vi "refNewton Ralphson Zero Finder.vi"   [LabVIEW 2012, in "NI_Gmath.lvlib"]
uses:
  NI_Gmath.lvlib
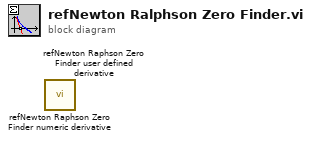
[diagram p0: block diagram]
diagram:
  n1 = call "refNewton Raphson Zero Finder numeric derivative.vi"() -> ()  [unwired: 8 in, 4 out]
  n2 = call "refNewton Raphson Zero Finder user defined derivative.vi"() -> ()  [unwired: 8 in, 4 out]
